vi "Test Request from TCP.vi"() -> ()   [LabVIEW 2020]
uses:
  HTTP Utils/Method.ctl
  lv-uri/URI/URI/URI.lvclass/URI.ctl
  lv-uri/URI/Build URI String.vi
  lv-uri/URI/Build Query String.vi
  HTTP Utils/Request/Request.lvclass
  lv-uri/URI/URI/URI.lvclass
  HTTP Utils/HTTP Utils.lvlib
panel:
  out "TTFB":dbl
  out "Error":errorcluster
  out "Body":string
  out "Headers":cluster{"Header":string, "Value":string}[](array[cluster])=[{"Header"="accept-encoding", "Value"="gzip, deflate"}, {"Header"="accept-language", "Value"="en-us"}, {"Header"="connection", "Value"="Keep-Alive"}, {"Header"="host", "Value"="www.tutorialspoint.com"}, {"Header"="user-agent", "Value"="Mozilla/4.0 (compatible; MSIE5.01; Windows NT)"}]
  out "Version String":string="HTTP/1.1"
  out "Method":T1
  out "Target":string="/hello.htm"
  in  "Listen Port":u16=36987
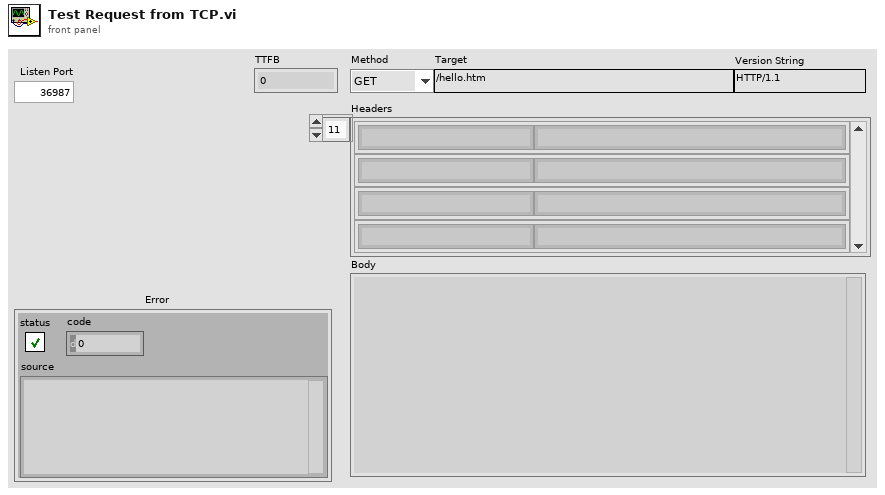
[diagram p1: front panel]
types:
  T1 = typedef "HTTP Utils.lvlib/Method.ctl" = enum16{"GET", "HEAD", "POST", "PUT", "DELETE", "CONNECT", "OPTIONS", "TRACE", "PATCH"}
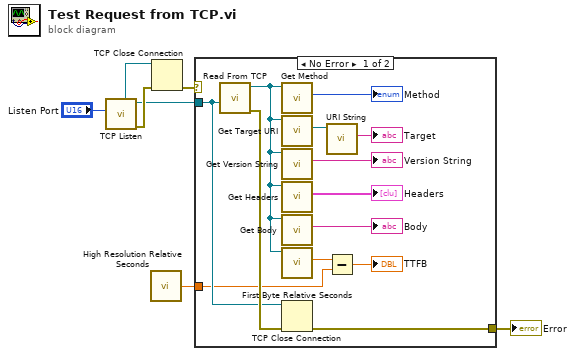
[diagram p0: block diagram]
diagram:
  n1 = call <vilib>:"TCP Listen.vi"("port"="Listen Port") -> ("error out"=w6:errorcluster, "connection ID"=w3:refnum<k5>, "listener ID"=w5:refnum<k5>)  [unwired: 6 in, 2 out]
  n2 = call <vilib>:"High Resolution Relative Seconds.vi"() -> ("relative seconds"=w1:dbl)
  n3 = TCP Close Connection(connection ID=w5, error in (no error)=w6) -> (error out=w4:errorcluster)  [unwired: 1 in, 1 out]
  n4 = case shown="No Error" w4 {
    selector: w4 -> [_ w21]
    tunnel: w3 -> [w13 _]
    tunnel: [w12 w21] -> w2
    tunnel: w1 -> [w11 _]
    frame No Error {
      n5 = call "Read From TCP.vi"("TCP Connection"=w13) -> ("error out"=w20:errorcluster, "Request out"=w9:refnum<class "Request.lvclass">)  [unwired: 9 in]
      n6 = call "Get Method.vi"("Request in"=w9) -> ("Method"=→"Method":T1)  [unwired: 8 in, 2 out]
      n7 = call "Get Target URI.vi"("Request in"=w9) -> ("Target URI"=w19:refnum<class "URI.lvclass">)  [unwired: 8 in, 2 out]
      n8 = call "Get Version String.vi"("Request in"=w9) -> ("Version String"=→"Version String":string)  [unwired: 8 in, 2 out]
      n9 = call "Get Headers.vi"("Request in"=w9) -> ("Headers"=→"Headers":cluster{"Header":string, "Value":string}[])  [unwired: 8 in, 2 out]
      n10 = call "Get Body.vi"("Request in"=w9) -> ("Body"=→"Body":string)  [unwired: 8 in, 2 out]
      n11 = call "First Byte Relative Seconds.vi"("Request in"=w9) -> ("First Byte Relative Seconds"=w10:dbl)  [unwired: 8 in, 2 out]
      n12 = TCP Close Connection(connection ID=w13, error in (no error)=w20) -> (error out=w12:errorcluster)  [unwired: 1 in, 1 out]
      n13 = call "URI String.vi"("URI in"=w19) -> ("URI String"=→"Target":string)  [unwired: 9 in, 1 out]
      n14 = Subtract(x=w10, y=w11) -> (x-y=→"TTFB":dbl)
    }
    frame Error {
    }
  }
  "Error" <- w2
